vi "Notifier_Driver.vi"(0 "Notification":bool, 2 "Notifier_Name":string, 11 "Error_In":errorcluster, 13 "Notifier_Operation_Select":T1=enum."Get_Notification_Status") -> (4 "Latest_Notification":bool, 15 "Error_Out":errorcluster)   [LabVIEW 2023]
doc: "Used to Create, Send, Receive and release the notifier."
uses:
  Controls/Notifier_Operation_Select.ctl
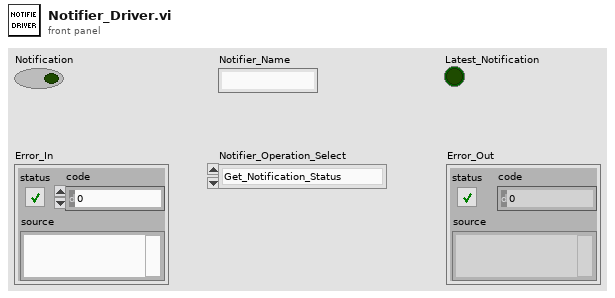
[diagram p1: front panel]
types:
  T1 = typedef "Notifier_Operation_Select.ctl" = enum16{"Obtain_Notification", "Send_Notification", "Get_Notification_Status", "Release_Notification"}
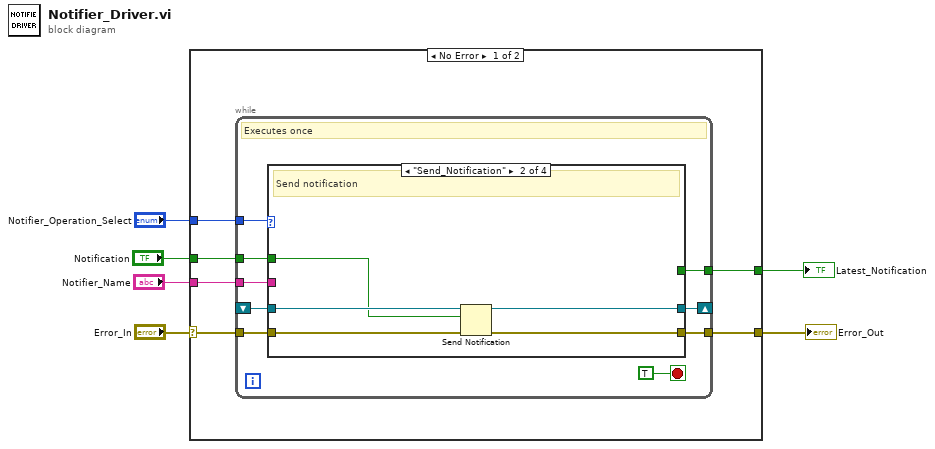
[diagram p0: block diagram]
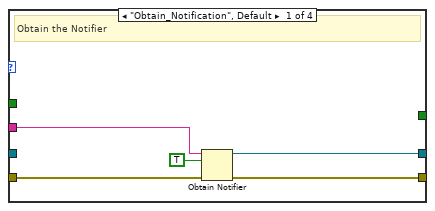
[diagram p2: hidden frame]
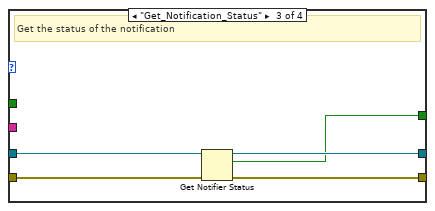
[diagram p3: hidden frame]
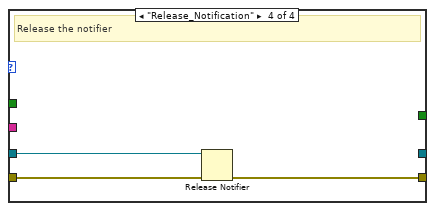
[diagram p4: hidden frame]
diagram:
  n1 = case shown="No Error" "Error_In" {
    selector: "Error_In" -> [w7 w40]
    tunnel: [w12 w40] -> w6
    tunnel: "Notifier_Name" -> [w11 _]
    tunnel: "Notification" -> [w10 _]
    tunnel: "Notifier_Operation_Select" -> [w9 _]
    tunnel: [w8 _] -> w2
    frame No Error {
      n2 = while {
        tunnel: w7 -> [w21]
        tunnel: [w19] -> w12
        tunnel: w11 -> [w18]
        shift-right: [w17] -> _
        shift-left: _ -> [w16]
        tunnel: w10 -> [w15]
        tunnel: w9 -> [w14]
        tunnel: [w13] -> w8
        stop <- TRUE stop-if-true
        # "Executes once"
        n3 = case shown="\"Send_Notification\"" w14 {
          tunnel: [w25 w30 w35 w38] -> w19
          tunnel: w21 -> [w26 w31 w36 w39]
          tunnel: w18 -> [w23 _ _ _]
          tunnel: [w22 w27 w33 _] -> w17
          tunnel: w16 -> [_ w29 w34 w37]
          tunnel: w15 -> [_ w28 _ _]
          tunnel: [_ _ w32 _] -> w13
          frame "Obtain_Notification", Default {
            # "Obtain the Notifier"
            n4 = Obtain Notifier(name (unnamed)=w23, notification data type=TRUE, error in (no error)=w26) -> (notifier out=w22:refnum<notifier>, error out=w25:errorcluster)  [unwired: 1 in, 1 out]
          }
          frame "Send_Notification" {
            # "Send notification"
            n5 = Send Notification(notification=w28, notifier=w29, error in (no error)=w31) -> (notifier out=w27:refnum<notifier>, error out=w30:errorcluster)
          }
          frame "Get_Notification_Status" {
            # "Get the status of the notification"
            n6 = Get Notifier Status(notifier=w34, error in (no error)=w36) -> (notifier out=w33:refnum<notifier>, current notification=w32:bool, error out=w35:errorcluster)  [unwired: 2 out]
          }
          frame "Release_Notification" {
            # "Release the notifier"
            n7 = Release Notifier(notifier=w37, error in (no error)=w39) -> (error out=w38:errorcluster)  [unwired: 1 in, 2 out]
          }
        }
      }
    }
    frame Error {
    }
  }
  "Error_Out" <- w6
  "Latest_Notification" <- w2
